vi "SaveControlValues.vi"(1 "file path":path, 2 "vi path":path) -> (0 "error out":errorcluster)   [LabVIEW 2011]
uses:
  <vilib>/Utility/config.llb/Write Key (String).vi
  <vilib>/Utility/config.llb/NI_LVConfig.lvlib
panel:
  out "Get All Control Values":T1(array[cluster])
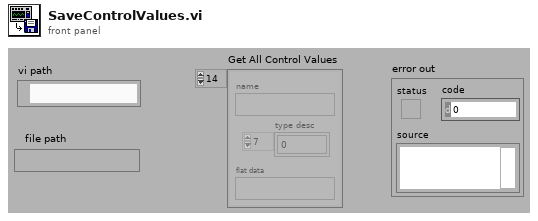
[diagram p1: front panel]
types:
  T1 = cluster{"name":string, "type desc":i16[], "flat data":string}[]
  T2 = typedef "NI_LVConfig.lvlib/Config Data RefNum.ctl" = refnum<k1>
  T3 = cluster{"name":string, "type desc":i16[], "flat data":string}
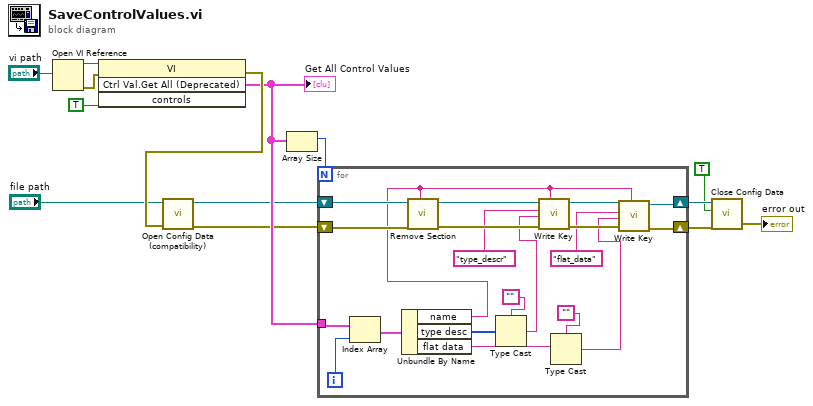
[diagram p0: block diagram]
diagram:
  n1 = Open VI Reference(vi path="vi path") -> (vi reference=w14:refnum<vi>, error out=w12:errorcluster)  [unwired: 5 in]
  n2 = invoke class="VI" method="Ctrl Val.Get All (Deprecated)"(reference=w14, error in=w12, "controls"=TRUE) -> (error out=w9:errorcluster, "Get All Control Values"=w6:T1)  [unwired: 1 in, 2 out]
  "Get All Control Values" <- w6
  n3 = call <vilib>:"Open Config Data (compatibility).vi"("error in (no error)"=w9, "configuration file path"="file path") -> ("error out"=w4:errorcluster, "refnum"=w5:T2)  [unwired: 7 in, 1 out]
  n4 = Array Size(array=w6) -> (size(s)=w7:i32)
  n5 = for {
    N: w7 -> [_]
    tunnel: w6 -> [w33]
    shift-right: [w22] -> w3
    shift-left: w5 -> [w31]
    shift-right: [w21] -> w2
    shift-left: w4 -> [w30]
    i -> [w32]
    n6 = Index Array(array=w33, index=w32) -> (element=w34:T3)
    n7 = Unbundle By Name(w34) -> ("name"=w20:string, "type desc"=w26:i16[], "flat data"=w16:string)
    n8 = call <vilib>:"Remove Section.vi"("section"=w20, "error in (no error)"=w30, "refnum"=w31) -> ("error out"=w28:errorcluster, "refnum out"=w29:T2)  [unwired: 6 in, 1 out]
    n9 = Type Cast(type="", x=w26) -> (*(type *) &x=w19:string)
    n10 = call-poly <vilib>:"Write Key.vi"("section"=w20, "error in (no error)"=w28, "value"=w19, "key"="type_descr", "refnum"=w29) -> ("error out"=w24:errorcluster, "refnum out"=w25:T2)  [unwired: 4 in, 1 out]
    n11 = Type Cast(type="", x=w16) -> (*(type *) &x=w15:string)
    n12 = call-poly <vilib>:"Write Key.vi"("section"=w20, "error in (no error)"=w24, "value"=w15, "key"="flat_data", "refnum"=w25) -> ("error out"=w21:errorcluster, "refnum out"=w22:T2)  [unwired: 4 in, 1 out]
  }
  n13 = call <vilib>:"Close Config Data.vi"("error in (no error)"=w2, "write file if changed (T)"=TRUE ("write configuration file? (T)"), "refnum"=w3) -> ("error out"=→"error out":errorcluster)  [unwired: 7 in, 1 out]
